vi "ge_EnblHiLite.vi"(8 "error in":errorcluster, 9 "CellSize":T3, 10 "ActiveCellPos":T2, 11 "FP Ctrl":T1) -> (0 "error out":errorcluster, 1 "Discard?":bool)   [LabVIEW 2012]
uses:
  <vilib>/Utility/miscctls.llb/LVBoundsTypeDef.ctl
  <vilib>/Utility/miscctls.llb/LVPositionTypeDef.ctl
  Custom Ctrls/ge_FPCtrlRefLabel.ctl
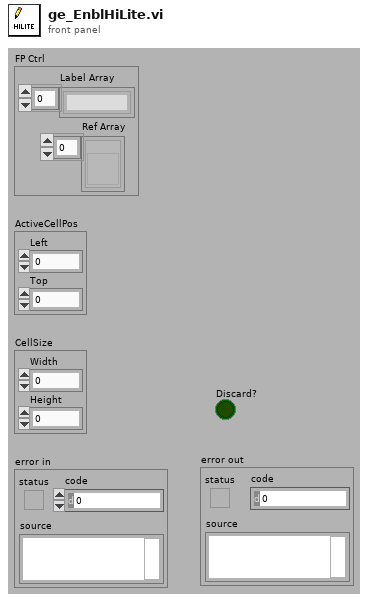
[diagram p1: front panel]
types:
  T1 = typedef "ge_FPCtrlRefLabel.ctl" = cluster{"Label Array":string[], "Ref Array":refnum<vi>[]}
  T2 = typedef "LVPositionTypeDef.ctl" = cluster{"Left":i32, "Top":i32}
  T3 = typedef "LVBoundsTypeDef.ctl" = cluster{"Width":u32, "Height":u32}
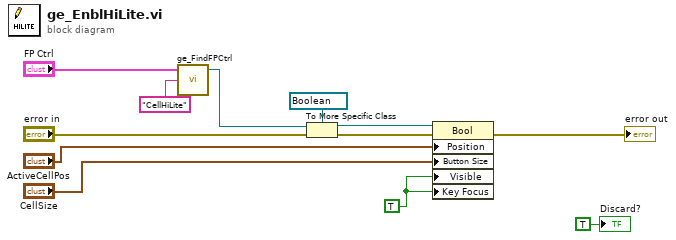
[diagram p0: block diagram]
diagram:
  w2 = TRUE ("Visible")
  n1 = call "ge_FindFPCtrl.vi"("Ctrl Name"="CellHiLite" ("Name"), "FP Ctrl"="FP Ctrl") -> ("Ctrl Ref"=w6:refnum<vi>)  [unwired: 3 in]
  n2 = To More Specific Class(target class=refnum<vi> refnum ("CellHiLite"), reference=w6, error in="error in") -> (specific class reference=w5:refnum<vi>, error out=w4:errorcluster)
  n3 = property class="Bool"(reference=w5, error in=w4, "Position"="ActiveCellPos", "Button Size"="CellSize", "Visible"=w2, "Key Focus"=w2) -> (error out=→"error out":errorcluster)  [unwired: 1 out]
  "Discard?" <- TRUE ("Discard?")
